vi "get_19052_PA_step_test_time.vi"(8 "error in (no error)":errorcluster, 10 "step":u16=1 min=1 max=99 step=1, 11 "VISA resource in":refnum<visa-resource-name>) -> (0 "error out":errorcluster, 2 "PA total time":string, 3 "VISA resource out":refnum<visa-resource-name>)   [LabVIEW 2015]
doc: "This VI retrieves the test TIME of the selected step and mode."
panel:
  # "Get 19052 PA test time"
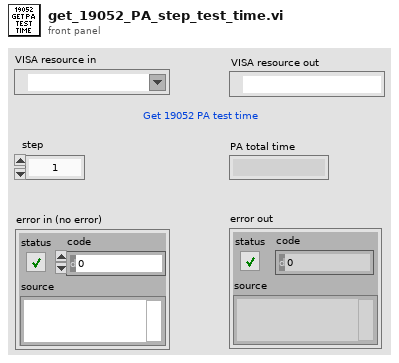
[diagram p1: front panel]
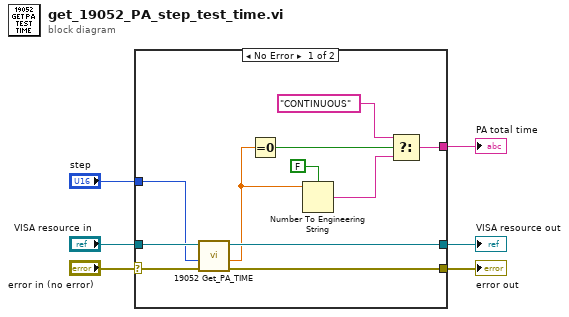
[diagram p0: block diagram]
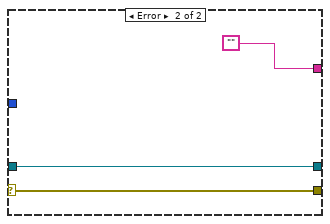
[diagram p2: hidden frame]
diagram:
  n1 = case shown="No Error" "error in (no error)" {
    selector: "error in (no error)" -> [w7 w20]
    tunnel: [w17 w20] -> w6
    tunnel: "VISA resource in" -> [w16 w19]
    tunnel: [w15 w19] -> w4
    tunnel: "step" -> [w14 _]
    tunnel: [w8 ""] -> w2
    frame No Error {
      n2 = call "19052 Get_PA_TIME.vi"("error in (no error)"=w7, "Step"=w14, "VISA resource in"=w16) -> ("error out"=w17:errorcluster, "Pause Time"=w11:dbl, "VISA resource out"=w15:refnum<visa-resource-name>)  [unwired: 6 in]
      n3 = Equal To 0?(x=w11) -> (x = 0?=w13:bool)
      n4 = Number To Engineering String(1:FALSE ("use system decimal point (T)"), 4:w11) -> (0:w9:string)  [unwired: 2 in]
      n5 = Select(t="CONTINUOUS", s=w13, f=w9) -> (s? t:f=w8:string)
    }
    frame Error {
    }
  }
  "error out" <- w6
  "VISA resource out" <- w4
  "PA total time" <- w2
